vi "StartVideo NewWindow.vi"(0 "VLC Variables In":T1, 1 "PictureBox":refnum<k24>(container), 9 "Media Source":string="dshow://", 11 "error in (no error)":errorcluster, 12 "Script":string) -> (4 "VLC Variables Out":T1, 15 "error out":errorcluster)   [LabVIEW 2012]
doc: "Set up all option to start streaming video from the webcam"
uses:
  Controls-Webcam/VLC Var.ctl
  System.Windows.Forms
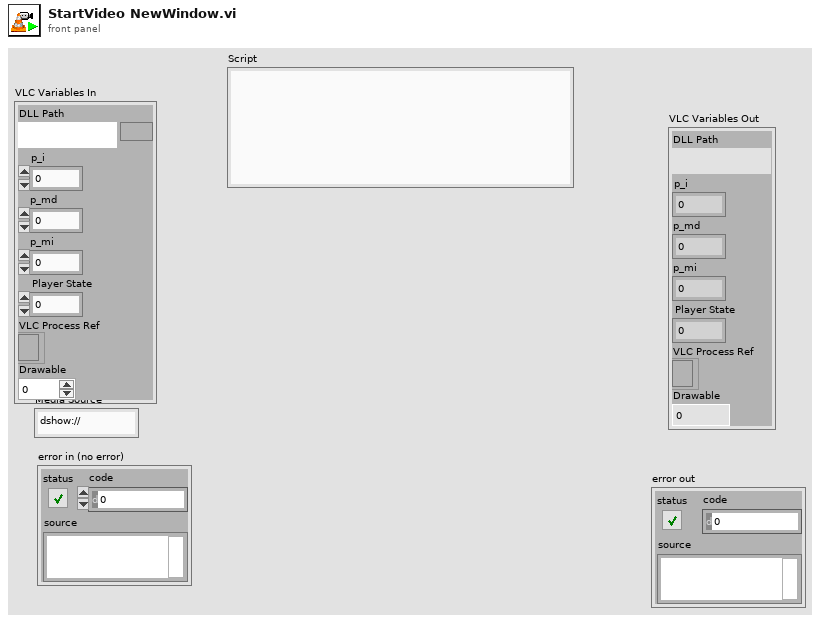
[diagram p1: front panel]
types:
  T1 = typedef "VLC Var.ctl" = cluster{"DLL Path":path, "p_i":i32, "p_md":i32, "p_mi":i32, "Player State":i32, "VLC Process Ref":refnum<k24>, "Drawable":i32}
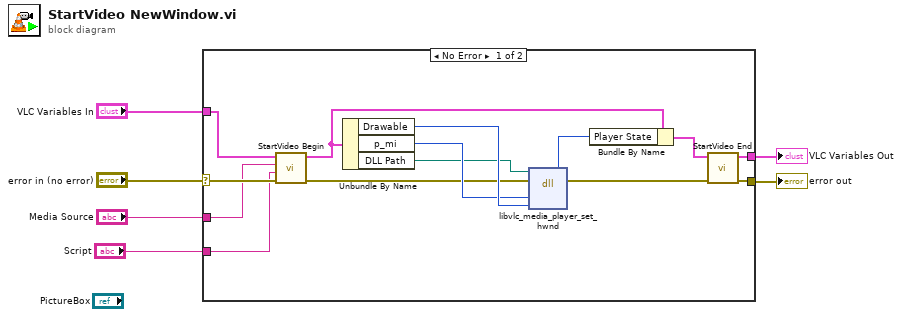
[diagram p0: block diagram]
diagram:
  n1 = case shown="No Error" "error in (no error)" {
    selector: "error in (no error)" -> [w9 w22]
    tunnel: "Media Source" -> [w8 _]
    tunnel: [w18 w21] -> w5
    tunnel: [w16 w22] -> w4
    tunnel: "Script" -> [w7 _]
    tunnel: "VLC Variables In" -> [w10 w21]
    frame No Error {
      n2 = call "StartVideo Begin.vi"("error in (no error)"=w9, "Script"=w7, "Media Source"=w8, "VLC Variables In in"=w10) -> ("error out"=w11:errorcluster, "VLC Variables In out"=w12:T1)  [unwired: 6 in]
      n3 = Unbundle By Name(w12) -> ("Drawable"=w15:i32, "p_mi"=w14:i32, "DLL Path"=w13:path)
      n4 = dll-call lib="C:/Program Files (x86)/VideoLAN/VLC/libvlc.dll" fn="libvlc_media_player_set_hwnd"(path in=w13, error in=w11, "p_mi"=w14, "handle"=w15) -> (error out=w19:errorcluster, "p_mi"=w20:i32)  [unwired: 3 in, 1 out]
      n5 = Bundle By Name(cluster=w12, "Player State"=w20) -> (w17:T1)
      n6 = call "StartVideo End.vi"("error in (no error)"=w19, "VLC Variables In in"=w17) -> ("error out"=w16:errorcluster, "VLC Variables In out"=w18:T1)  [unwired: 8 in]
    }
    frame Error {
    }
  }
  "error out" <- w4
  "VLC Variables Out" <- w5
